vi "CameraList.vi"(2 "error in":errorcluster, 3 "node":string) -> (0 "error out":errorcluster, 1 "Cameras List":T1)   [LabVIEW 2010]
uses:
  ROS/Code/SubVIs/_ROSDirection.ctl
  ROS/Code/Console/Servers/ServerSubs/TopicDef.ctl
panel:
  out "Reply":string
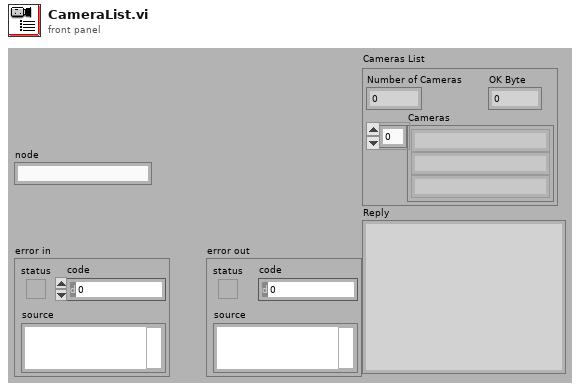
[diagram p1: front panel]
types:
  T1 = cluster{"Number of Cameras":i32, "Cameras":string[], "OK Byte":u8}
  T2 = typedef "TopicDef.ctl" = cluster{"Topic":string, "Type":string, "Action":T3, "Update (ms)":u16, "write queue":u16}
  T3 = typedef "_ROSDirection.ctl" = enum16{"Node", "Publisher", "Subscriber", "Service Client"}
  T4 = typedef "_ROSControl.ctl" = cluster{"topic port":u16, "Node":string, "topic":string, "type":string, "node port":u32, "error ":errorcluster, "Direction":T3, "APIs":string[], "Update (ms)":u16, "write queue":u16}
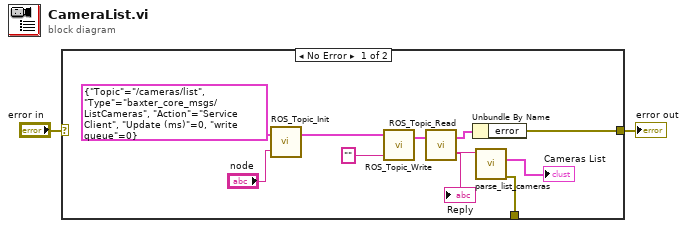
[diagram p0: block diagram]
diagram:
  n1 = case shown="No Error" "error in" {
    selector: "error in" -> [_ w13]
    tunnel: [w12 w13] -> w2
    tunnel: [w4 _] -> _
    frame No Error {
      n2 = call "ROS_Topic_Init.vi"("node"="node", "Definitions"=T2 {"Topic"="/cameras/list", "Type"="baxter_core_msgs/ListCameras", "Action"=enum."Service Client", "Update (ms)"=0, "write queue"=0}) -> ("ROS out"=w10:T4)  [unwired: 1 in]
      n3 = call "ROS_Topic_Write.vi"("Msg in"="", "ROS in"=w10) -> ("ROS out"=w9:T4)  [unwired: 2 in]
      n4 = call "ROS_Topic_Read.vi"("ROS in"=w9) -> ("Reply"=w6:string, "ROS out"=w8:T4)  [unwired: 1 in]
      "Reply" <- w6
      n5 = Unbundle By Name(w8) -> ("error"=w12:errorcluster)
      n6 = call "parse_list_cameras.vi"("msg in"=w6) -> ("error out"=w4:errorcluster, "Cameras List"=→"Cameras List":T1)  [unwired: 4 in, 1 out]
    }
    frame Error {
    }
  }
  "error out" <- w2
